vi "Autonomous State Machine.vi"   [LabVIEW 2014]
doc: "This VI is called when autonomous begins, and will automatically be terminated when autonomous ends. You can carry out timed or sensor driven robot movement independently without needing to return to the caller."
uses:
  <vilib>/Rock Robotics/WPI/RobotDrive/WPI_RobotDriveGetSetRefNum.vi
panel:
  # "Be sure to right-click and choose Data Operations>>Make Current Value default if you want to save the array values with the VI"
types:
  T1 = typedef "WPI_MotorControlDeviceRef.ctl" = cluster{"DeviceStatus":errorcluster, "Type":T2, "PWM":cluster{"Controller":T3, "PWM Channel":T4, "DeadBand":T5}, "CAN":cluster{"Device Number":u8, "Control Mode":T6, "Semaphore":T7, "Max Vout":dbl, "TalonSRX Control Mode":T8}, "Invert":bool, "TransformRef":T9, "InvTransformRef":T9}
  T2 = typedef "WPI_MotorControlType.ctl" = enum16{"PWM", "CAN", "CANTalonSRX"}
  T3 = typedef "FPGA_TypedefDigitalModule.ctl" = enum16{"Controller 1"}
  T4 = typedef "FPGA_DIOPWMChannel.ctl" = enum8{"PWM 0", "PWM 1", "PWM 2", "PWM 3", "PWM 4", "PWM 5", "PWM 6", "PWM 7", "PWM 8", "PWM 9", "PWM MXP 0", "PWM MXP 1", "PWM MXP 2", "PWM MXP 3", "PWM MXP 4", "PWM MXP 5", "PWM MXP 6", "PWM MXP 7", "PWM MXP 8", "PWM MXP 9", "Invalid"}
  T5 = typedef "WPI_PWMDeadband.ctl" = cluster{"Name":string, "maxPositivePwm":i32, "minPositivePwm":i32, "centerPwm":i32, "maxNegativePwm":i32, "minNegativePwm":i32, "angularRange":u16}
  T6 = typedef "WPI_CANJaguar_ControlMode.ctl" = enum8{"Percent VBus", "Current", "Speed", "Position", "Voltage"}
  T7 = typedef "Semaphore RefNum" = refnum<k1>
  T8 = typedef "WPI_CANTalonSRX_APIControlMode.ctl" = enum8{"Percent VBus", "Speed", "Position", "Slave", "Unchanged / Invalid"}
  T9 = typedef "WPI_PWMTransform_ConPane.ctl" = refnum<vi>
  T10 = typedef "WPI_DigitalInputDevRef.ctl" = cluster{"DevStatus":errorcluster, "DIO Channel":T11, "Controller":T3}
  T11 = typedef "FPGA_DIOChannel.ctl" = enum8{"DIO 0", "DIO 1", "DIO 2", "DIO 3", "DIO 4", "DIO 5", "DIO 6", "DIO 7", "DIO 8", "DIO 9", "DIO MXP 0", "DIO MXP 1", "DIO MXP 2", "DIO MXP 3", "DIO MXP 4", "DIO MXP 5", "DIO MXP 6", "DIO MXP 7", "DIO MXP 8", "DIO MXP 9", "DIO MXP 10", "DIO MXP 11", "DIO MXP 12", "DIO MXP 13", "DIO MXP 14", "DIO MXP 15", "Invalid"}
  T12 = typedef "WPI_RobotDriveDevRef.ctl" = cluster{"DevStatus":errorcluster, "Motors[]":T1[], "Square Inputs":bool, "Max Output":dbl}
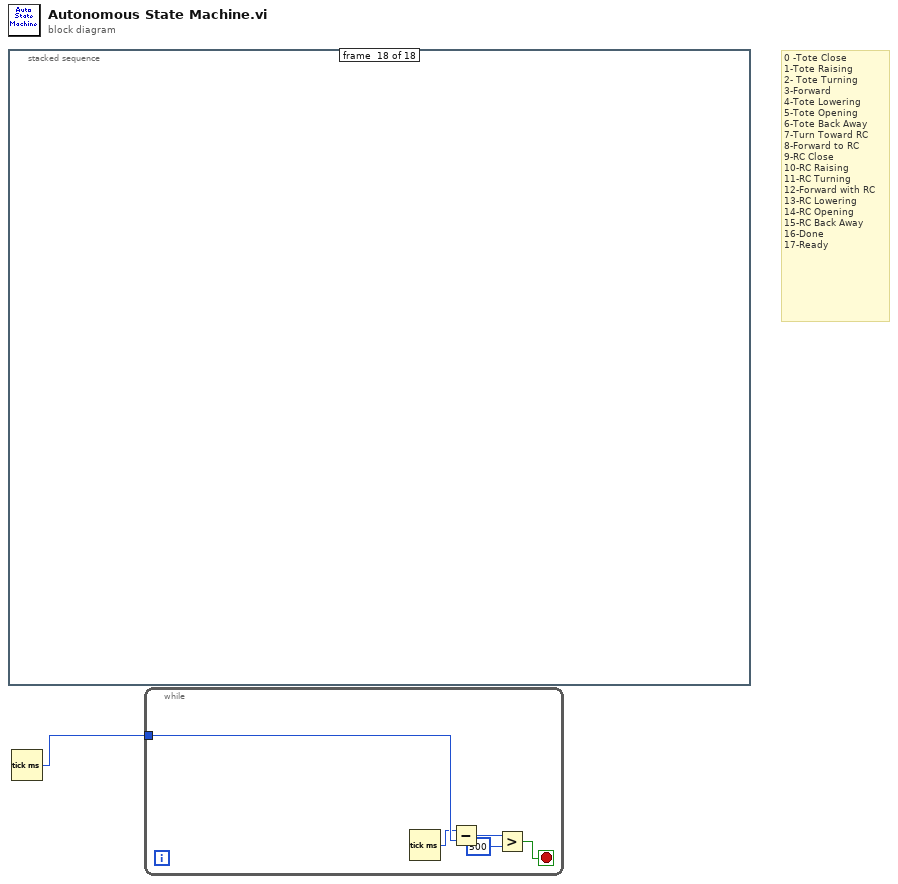
[diagram p0: block diagram]
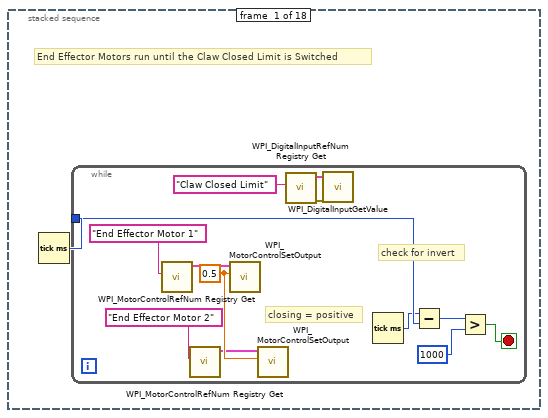
[diagram p2: hidden frame]
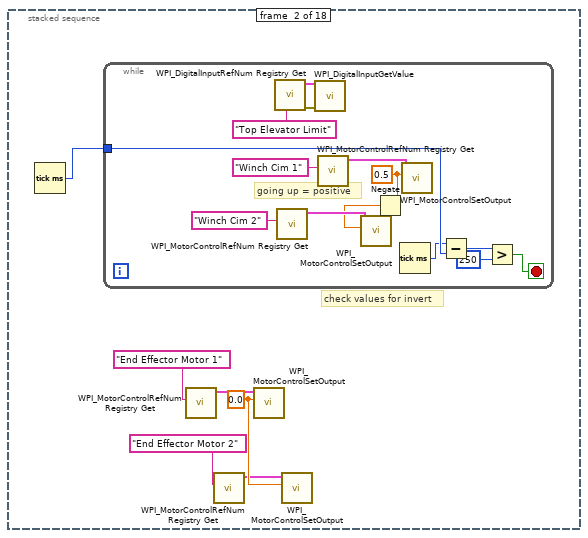
[diagram p3: hidden frame]
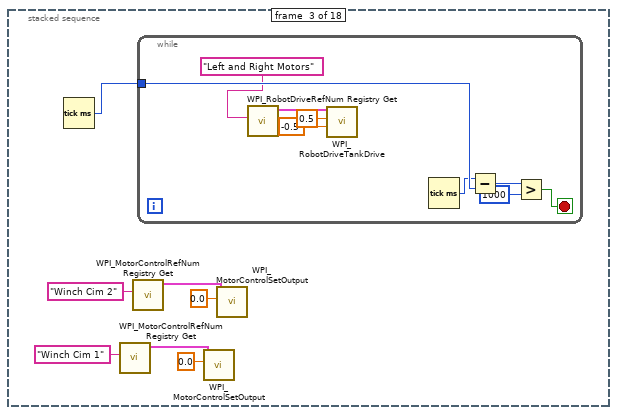
[diagram p4: hidden frame]
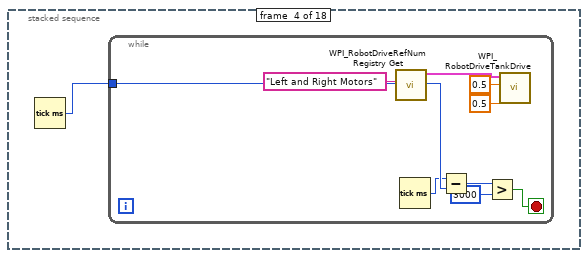
[diagram p5: hidden frame]
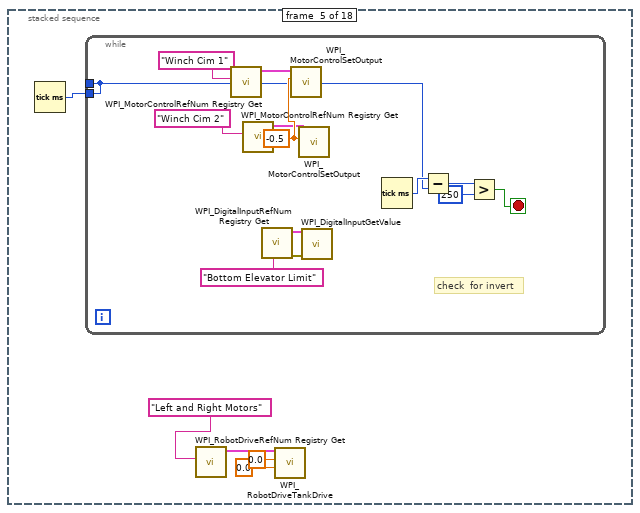
[diagram p6: hidden frame]
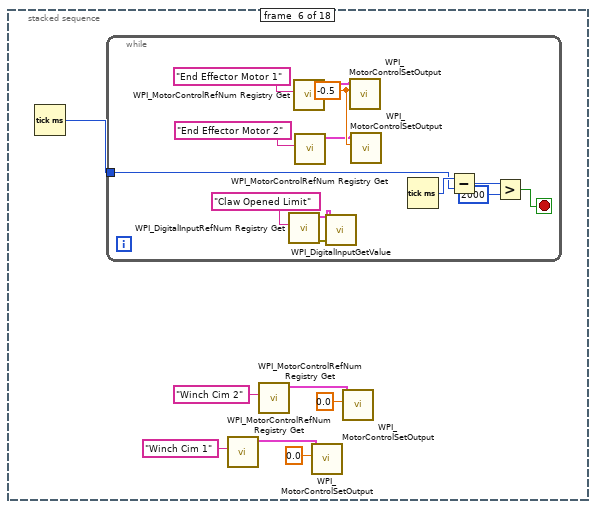
[diagram p7: hidden frame]
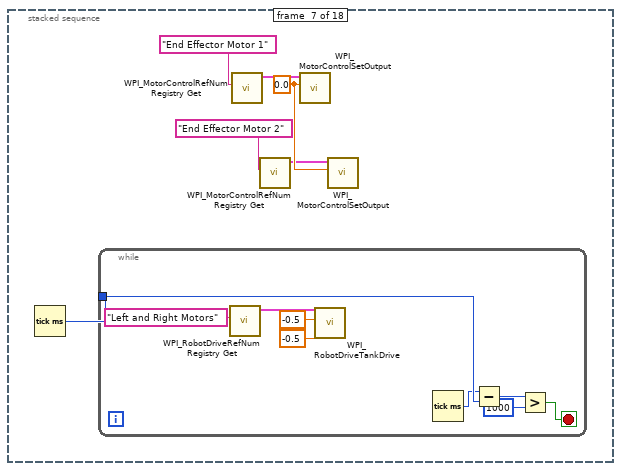
[diagram p8: hidden frame]
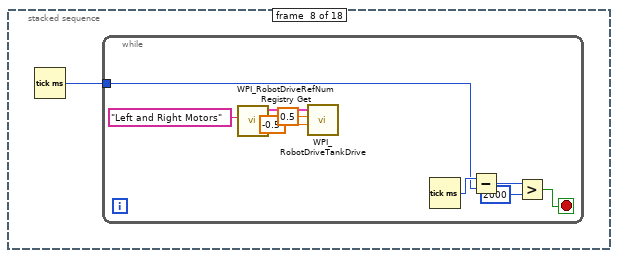
[diagram p9: hidden frame]
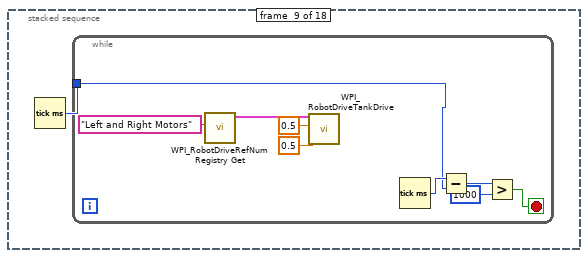
[diagram p10: hidden frame]
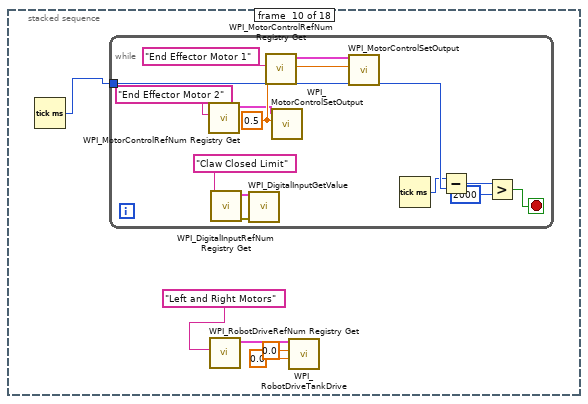
[diagram p11: hidden frame]
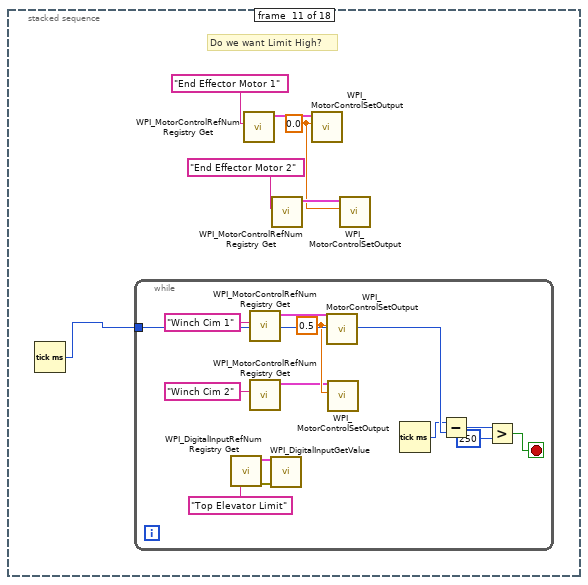
[diagram p12: hidden frame]
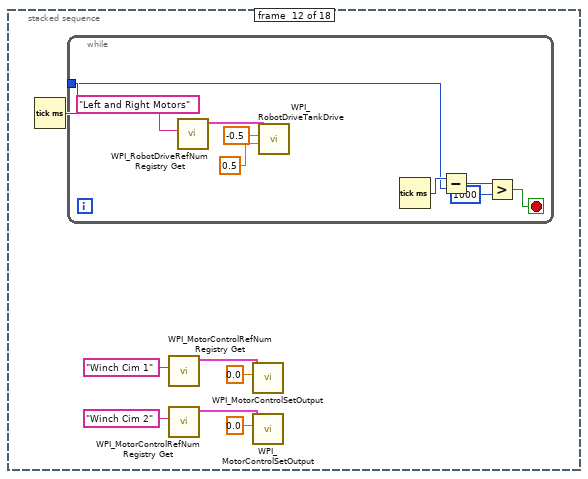
[diagram p13: hidden frame]
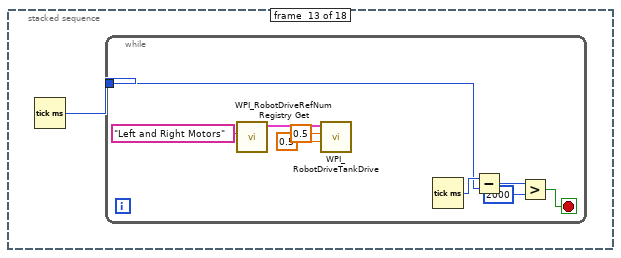
[diagram p14: hidden frame]
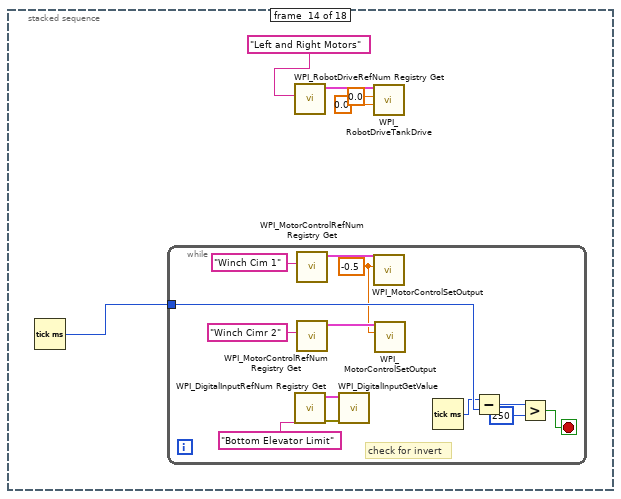
[diagram p15: hidden frame]
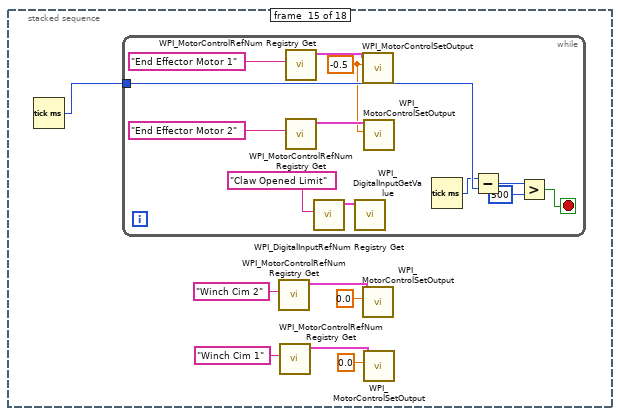
[diagram p16: hidden frame]
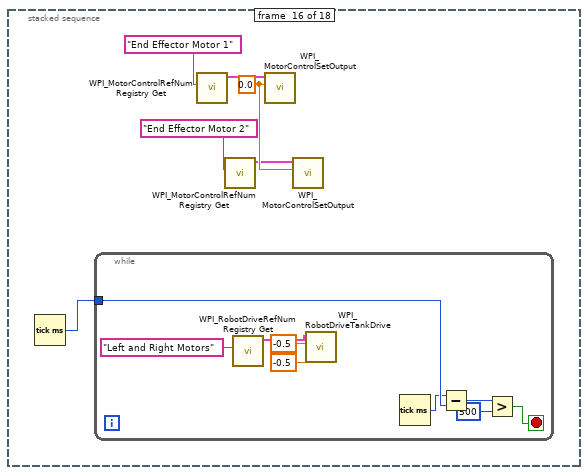
[diagram p17: hidden frame]
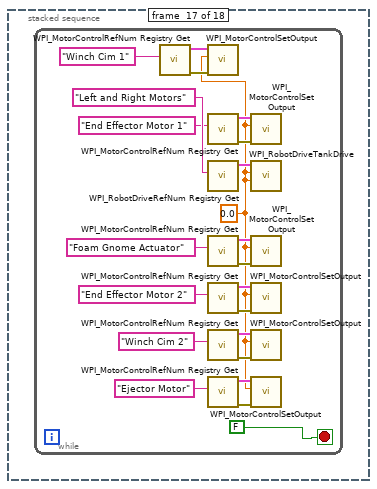
[diagram p18: hidden frame]
diagram:
  # "0 -Tote Close\n1-Tote Raising\n2- Tote Turning\n3-Forward\n4-Tote Lowering\n5-Tote Opening\n6-Tote Back Away\n7-Turn Toward RC\n8-Forward to RC\n9-RC Close\n10-RC Raising\n11-RC Turning\n12-Forward with RC\n13-RC Lowering\n14-RC Opening\n15-RC Back Away\n16-Done\n17-Ready"
  n1 = stacked-sequence {
    frame #0 {
      # "End Effector Motors run until the Claw Closed Limit is Switched"
      n2 = Tick Count (ms)() -> (millisecond timer value=w2:u32)
      n3 = while {
        tunnel: w2 -> [w12]
        stop <- w13 stop-if-true
        w9 = 0.5 ("Output")
        # "closing = positive"
        # "check for invert"
        n4 = call <vilib>:"WPI_MotorControlRefNum Registry Get.vi"("refnum name"="End Effector Motor 1") -> ("MotorControlDevRef"=w6:T1)  [unwired: 9 in, 1 out]
        n5 = call <vilib>:"WPI_MotorControlRefNum Registry Get.vi"("refnum name"="End Effector Motor 2") -> ("MotorControlDevRef"=w8:T1)  [unwired: 9 in, 1 out]
        n6 = call <vilib>:"WPI_MotorControlSetOutput.vi"("Output"=w9, "MotorControlDevRef"=w6) -> ()  [unwired: 7 in, 3 out]
        n7 = call <vilib>:"WPI_MotorControlSetOutput.vi"("Output"=w9, "MotorControlDevRef"=w8) -> ()  [unwired: 7 in, 3 out]
        n8 = call <vilib>:"WPI_DigitalInputRefNum Registry Get.vi"("refnum name"="Claw Closed Limit") -> ("error out"=w4:errorcluster, "DigitalInputDevRef"=w3:T10)  [unwired: 9 in]
        n9 = call <vilib>:"WPI_DigitalInputGetValue.vi"("error in (no error)"=w4, "DigitalInputDevRef"=w3) -> ()  [unwired: 7 in, 3 out]
        n10 = Tick Count (ms)() -> (millisecond timer value=w11:u32)
        n11 = Subtract(x=w11, y=w12) -> (x-y=w15:u32)
        n12 = Greater?(x=w15, y=u32 1000) -> (0:w13:bool)
      }
    }
    frame #1 {
      w19 = 0.0 ("Output")
      # "check values for invert"
      n13 = Tick Count (ms)() -> (millisecond timer value=w21:u32)
      n14 = while {
        tunnel: w21 -> [w26]
        stop <- w27 stop-if-true
        w31 = 0.5 ("Output")
        # "going up = positive"
        n15 = call <vilib>:"WPI_DigitalInputRefNum Registry Get.vi"("refnum name"="Top Elevator Limit") -> ("error out"=w23:errorcluster, "DigitalInputDevRef"=w22:T10)  [unwired: 9 in]
        n16 = call <vilib>:"WPI_MotorControlRefNum Registry Get.vi"("refnum name"="Winch Cim 2") -> ("MotorControlDevRef"=w33:T1)  [unwired: 9 in, 1 out]
        n17 = call <vilib>:"WPI_DigitalInputGetValue.vi"("error in (no error)"=w23, "DigitalInputDevRef"=w22) -> ()  [unwired: 7 in, 3 out]
        n18 = call <vilib>:"WPI_MotorControlRefNum Registry Get.vi"("refnum name"="Winch Cim 1") -> ("MotorControlDevRef"=w35:T1)  [unwired: 9 in, 1 out]
        n19 = Negate(x=w31) -> (-x=w30:dbl)
        n20 = call <vilib>:"WPI_MotorControlSetOutput.vi"("Output"=w30, "MotorControlDevRef"=w33) -> ()  [unwired: 7 in, 3 out]
        n21 = Tick Count (ms)() -> (millisecond timer value=w25:u32)
        n22 = call <vilib>:"WPI_MotorControlSetOutput.vi"("Output"=w31, "MotorControlDevRef"=w35) -> ()  [unwired: 7 in, 3 out]
        n23 = Subtract(x=w25, y=w26) -> (x-y=w29:u32)
        n24 = Greater?(x=w29, y=u32 250) -> (0:w27:bool)
      }
      n25 = call <vilib>:"WPI_MotorControlRefNum Registry Get.vi"("refnum name"="End Effector Motor 1") -> ("MotorControlDevRef"=w16:T1)  [unwired: 9 in, 1 out]
      n26 = call <vilib>:"WPI_MotorControlRefNum Registry Get.vi"("refnum name"="End Effector Motor 2") -> ("MotorControlDevRef"=w18:T1)  [unwired: 9 in, 1 out]
      n27 = call <vilib>:"WPI_MotorControlSetOutput.vi"("Output"=w19, "MotorControlDevRef"=w16) -> ()  [unwired: 7 in, 3 out]
      n28 = call <vilib>:"WPI_MotorControlSetOutput.vi"("Output"=w19, "MotorControlDevRef"=w18) -> ()  [unwired: 7 in, 3 out]
    }
    frame #2 {
      n29 = Tick Count (ms)() -> (millisecond timer value=w42:u32)
      n30 = call <vilib>:"WPI_MotorControlRefNum Registry Get.vi"("refnum name"="Winch Cim 1") -> ("MotorControlDevRef"=w37:T1)  [unwired: 9 in, 1 out]
      n31 = call <vilib>:"WPI_MotorControlRefNum Registry Get.vi"("refnum name"="Winch Cim 2") -> ("MotorControlDevRef"=w40:T1)  [unwired: 9 in, 1 out]
      n32 = while {
        tunnel: w42 -> [w48]
        stop <- w49 stop-if-true
        n33 = call <vilib>:"WPI_RobotDriveRefNum Registry Get.vi"("refnum name"="Left and Right Motors") -> ("RobotDriveDevRef"=w46:T12)  [unwired: 9 in, 1 out]
        n34 = call <vilib>:"WPI_RobotDriveTankDrive.vi"("Right axis value"=-0.5, "Left axis value"=0.5, "RobotDriveDevRef"=w46) -> ()  [unwired: 6 in, 3 out]
        n35 = Tick Count (ms)() -> (millisecond timer value=w47:u32)
        n36 = Subtract(x=w47, y=w48) -> (x-y=w51:u32)
        n37 = Greater?(x=w51, y=u32 1000) -> (0:w49:bool)
      }
      n38 = call <vilib>:"WPI_MotorControlSetOutput.vi"("Output"=0.0, "MotorControlDevRef"=w37) -> ()  [unwired: 7 in, 3 out]
      n39 = call <vilib>:"WPI_MotorControlSetOutput.vi"("Output"=0.0, "MotorControlDevRef"=w40) -> ()  [unwired: 7 in, 3 out]
    }
    frame #3 {
      n40 = Tick Count (ms)() -> (millisecond timer value=w52:u32)
      n41 = while {
        tunnel: w52 -> [w58]
        stop <- w59 stop-if-true
        n42 = call <vilib>:"WPI_RobotDriveRefNum Registry Get.vi"("refnum name"="Left and Right Motors") -> ("RobotDriveDevRef"=w56:T12)  [unwired: 9 in, 1 out]
        n43 = Tick Count (ms)() -> (millisecond timer value=w57:u32)
        n44 = Subtract(x=w57, y=w58) -> (x-y=w61:u32)
        n45 = Greater?(x=w61, y=u32 3000) -> (0:w59:bool)
        n46 = call <vilib>:"WPI_RobotDriveTankDrive.vi"("Right axis value"=0.5, "Left axis value"=0.5, "RobotDriveDevRef"=w56) -> ()  [unwired: 6 in, 3 out]
      }
    }
    frame #4 {
      n47 = Tick Count (ms)() -> (millisecond timer value=w66:u32)
      n48 = while {
        tunnel: [w70] -> _
        tunnel: w66 -> [w70]
        stop <- w77 stop-if-true
        w75 = -0.5 ("Output")
        # "check  for invert"
        n49 = call <vilib>:"WPI_MotorControlRefNum Registry Get.vi"("refnum name"="Winch Cim 1") -> ("MotorControlDevRef"=w73:T1)  [unwired: 9 in, 1 out]
        n50 = call <vilib>:"WPI_MotorControlRefNum Registry Get.vi"("refnum name"="Winch Cim 2") -> ("MotorControlDevRef"=w74:T1)  [unwired: 9 in, 1 out]
        n51 = call <vilib>:"WPI_DigitalInputRefNum Registry Get.vi"("refnum name"="Bottom Elevator Limit") -> ("error out"=w68:errorcluster, "DigitalInputDevRef"=w67:T10)  [unwired: 9 in]
        n52 = call <vilib>:"WPI_MotorControlSetOutput.vi"("Output"=w75, "MotorControlDevRef"=w73) -> ()  [unwired: 7 in, 3 out]
        n53 = call <vilib>:"WPI_MotorControlSetOutput.vi"("Output"=w75, "MotorControlDevRef"=w74) -> ()  [unwired: 7 in, 3 out]
        n54 = call <vilib>:"WPI_DigitalInputGetValue.vi"("error in (no error)"=w68, "DigitalInputDevRef"=w67) -> ()  [unwired: 7 in, 3 out]
        n55 = Tick Count (ms)() -> (millisecond timer value=w76:u32)
        n56 = Subtract(x=w76, y=w70) -> (x-y=w79:u32)
        n57 = Greater?(x=w79, y=u32 250) -> (0:w77:bool)
      }
      n58 = call <vilib>:"WPI_RobotDriveRefNum Registry Get.vi"("refnum name"="Left and Right Motors") -> ("RobotDriveDevRef"=w65:T12)  [unwired: 9 in, 1 out]
      n59 = call <vilib>:"WPI_RobotDriveTankDrive.vi"("Right axis value"=0.0, "Left axis value"=0.0, "RobotDriveDevRef"=w65) -> ()  [unwired: 6 in, 3 out]
    }
    frame #5 {
      n60 = Tick Count (ms)() -> (millisecond timer value=w86:u32)
      n61 = while {
        tunnel: w86 -> [w90]
        stop <- w97 stop-if-true
        w95 = -0.5 ("Output")
        n62 = call <vilib>:"WPI_DigitalInputRefNum Registry Get.vi"("refnum name"="Claw Opened Limit") -> ("error out"=w88:errorcluster, "DigitalInputDevRef"=w89:T10)  [unwired: 9 in]
        n63 = call <vilib>:"WPI_MotorControlRefNum Registry Get.vi"("refnum name"="End Effector Motor 1") -> ("MotorControlDevRef"=w92:T1)  [unwired: 9 in, 1 out]
        n64 = call <vilib>:"WPI_MotorControlRefNum Registry Get.vi"("refnum name"="End Effector Motor 2") -> ("MotorControlDevRef"=w94:T1)  [unwired: 9 in, 1 out]
        n65 = call <vilib>:"WPI_DigitalInputGetValue.vi"("error in (no error)"=w88, "DigitalInputDevRef"=w89) -> ()  [unwired: 7 in, 3 out]
        n66 = call <vilib>:"WPI_MotorControlSetOutput.vi"("Output"=w95, "MotorControlDevRef"=w92) -> ()  [unwired: 7 in, 3 out]
        n67 = call <vilib>:"WPI_MotorControlSetOutput.vi"("Output"=w95, "MotorControlDevRef"=w94) -> ()  [unwired: 7 in, 3 out]
        n68 = Tick Count (ms)() -> (millisecond timer value=w96:u32)
        n69 = Subtract(x=w96, y=w90) -> (x-y=w99:u32)
        n70 = Greater?(x=w99, y=u32 2000) -> (0:w97:bool)
      }
      n71 = call <vilib>:"WPI_MotorControlRefNum Registry Get.vi"("refnum name"="Winch Cim 1") -> ("MotorControlDevRef"=w81:T1)  [unwired: 9 in, 1 out]
      n72 = call <vilib>:"WPI_MotorControlRefNum Registry Get.vi"("refnum name"="Winch Cim 2") -> ("MotorControlDevRef"=w84:T1)  [unwired: 9 in, 1 out]
      n73 = call <vilib>:"WPI_MotorControlSetOutput.vi"("Output"=0.0, "MotorControlDevRef"=w81) -> ()  [unwired: 7 in, 3 out]
      n74 = call <vilib>:"WPI_MotorControlSetOutput.vi"("Output"=0.0, "MotorControlDevRef"=w84) -> ()  [unwired: 7 in, 3 out]
    }
    frame #6 {
      w103 = 0.0 ("Output")
      n75 = Tick Count (ms)() -> (millisecond timer value=w105:u32)
      n76 = while {
        tunnel: w105 -> [w111]
        stop <- w112 stop-if-true
        n77 = call <vilib>:"WPI_RobotDriveRefNum Registry Get.vi"("refnum name"="Left and Right Motors") -> ("RobotDriveDevRef"=w109:T12)  [unwired: 9 in, 1 out]
        n78 = call <vilib>:"WPI_RobotDriveTankDrive.vi"("Right axis value"=-0.5, "Left axis value"=-0.5, "RobotDriveDevRef"=w109) -> ()  [unwired: 6 in, 3 out]
        n79 = Tick Count (ms)() -> (millisecond timer value=w110:u32)
        n80 = Subtract(x=w110, y=w111) -> (x-y=w114:u32)
        n81 = Greater?(x=w114, y=u32 1000) -> (0:w112:bool)
      }
      n82 = call <vilib>:"WPI_MotorControlRefNum Registry Get.vi"("refnum name"="End Effector Motor 1") -> ("MotorControlDevRef"=w100:T1)  [unwired: 9 in, 1 out]
      n83 = call <vilib>:"WPI_MotorControlRefNum Registry Get.vi"("refnum name"="End Effector Motor 2") -> ("MotorControlDevRef"=w102:T1)  [unwired: 9 in, 1 out]
      n84 = call <vilib>:"WPI_MotorControlSetOutput.vi"("Output"=w103, "MotorControlDevRef"=w100) -> ()  [unwired: 7 in, 3 out]
      n85 = call <vilib>:"WPI_MotorControlSetOutput.vi"("Output"=w103, "MotorControlDevRef"=w102) -> ()  [unwired: 7 in, 3 out]
    }
    frame #7 {
      n86 = Tick Count (ms)() -> (millisecond timer value=w115:u32)
      n87 = while {
        tunnel: w115 -> [w120]
        stop <- w122 stop-if-true
        n88 = call <vilib>:"WPI_RobotDriveRefNum Registry Get.vi"("refnum name"="Left and Right Motors") -> ("RobotDriveDevRef"=w119:T12)  [unwired: 9 in, 1 out]
        n89 = call <vilib>:"WPI_RobotDriveTankDrive.vi"("Right axis value"=-0.5, "Left axis value"=0.5, "RobotDriveDevRef"=w119) -> ()  [unwired: 6 in, 3 out]
        n90 = Tick Count (ms)() -> (millisecond timer value=w121:u32)
        n91 = Subtract(x=w121, y=w120) -> (x-y=w124:u32)
        n92 = Greater?(x=w124, y=u32 2000) -> (0:w122:bool)
      }
    }
    frame #8 {
      n93 = Tick Count (ms)() -> (millisecond timer value=w125:u32)
      n94 = while {
        tunnel: w125 -> [w130]
        stop <- w132 stop-if-true
        n95 = call <vilib>:"WPI_RobotDriveRefNum Registry Get.vi"("refnum name"="Left and Right Motors") -> ("RobotDriveDevRef"=w129:T12)  [unwired: 9 in, 1 out]
        n96 = call <vilib>:"WPI_RobotDriveTankDrive.vi"("Right axis value"=0.5, "Left axis value"=0.5, "RobotDriveDevRef"=w129) -> ()  [unwired: 6 in, 3 out]
        n97 = Tick Count (ms)() -> (millisecond timer value=w131:u32)
        n98 = Subtract(x=w131, y=w130) -> (x-y=w134:u32)
        n99 = Greater?(x=w134, y=u32 1000) -> (0:w132:bool)
      }
    }
    frame #9 {
      n100 = Tick Count (ms)() -> (millisecond timer value=w139:u32)
      n101 = while {
        tunnel: w139 -> [w149]
        stop <- w150 stop-if-true
        w147 = 0.5 ("Output")
        n102 = call <vilib>:"WPI_MotorControlRefNum Registry Get.vi"("refnum name"="End Effector Motor 2") -> ("MotorControlDevRef"=w144:T1)  [unwired: 9 in, 1 out]
        n103 = call <vilib>:"WPI_DigitalInputRefNum Registry Get.vi"("refnum name"="Claw Closed Limit") -> ("error out"=w141:errorcluster, "DigitalInputDevRef"=w142:T10)  [unwired: 9 in]
        n104 = call <vilib>:"WPI_DigitalInputGetValue.vi"("error in (no error)"=w141, "DigitalInputDevRef"=w142) -> ()  [unwired: 7 in, 3 out]
        n105 = call <vilib>:"WPI_MotorControlRefNum Registry Get.vi"("refnum name"="End Effector Motor 1") -> ("MotorControlDevRef"=w143:T1)  [unwired: 9 in, 1 out]
        n106 = call <vilib>:"WPI_MotorControlSetOutput.vi"("Output"=w147, "MotorControlDevRef"=w144) -> ()  [unwired: 7 in, 3 out]
        n107 = call <vilib>:"WPI_MotorControlSetOutput.vi"("Output"=w147, "MotorControlDevRef"=w143) -> ()  [unwired: 7 in, 3 out]
        n108 = Tick Count (ms)() -> (millisecond timer value=w148:u32)
        n109 = Subtract(x=w148, y=w149) -> (x-y=w152:u32)
        n110 = Greater?(x=w152, y=u32 2000) -> (0:w150:bool)
      }
      n111 = call <vilib>:"WPI_RobotDriveRefNum Registry Get.vi"("refnum name"="Left and Right Motors") -> ("RobotDriveDevRef"=w138:T12)  [unwired: 9 in, 1 out]
      n112 = call <vilib>:"WPI_RobotDriveTankDrive.vi"("Right axis value"=0.0, "Left axis value"=0.0, "RobotDriveDevRef"=w138) -> ()  [unwired: 6 in, 3 out]
    }
    frame #10 {
      w154 = 0.0 ("Output")
      # "Do we want Limit High?"
      n113 = Tick Count (ms)() -> (millisecond timer value=w158:u32)
      n114 = while {
        tunnel: w158 -> [w168]
        stop <- w169 stop-if-true
        w166 = 0.5 ("Output")
        n115 = call <vilib>:"WPI_DigitalInputRefNum Registry Get.vi"("refnum name"="Top Elevator Limit") -> ("error out"=w160:errorcluster, "DigitalInputDevRef"=w159:T10)  [unwired: 9 in]
        n116 = call <vilib>:"WPI_MotorControlRefNum Registry Get.vi"("refnum name"="Winch Cim 1") -> ("MotorControlDevRef"=w162:T1)  [unwired: 9 in, 1 out]
        n117 = call <vilib>:"WPI_MotorControlRefNum Registry Get.vi"("refnum name"="Winch Cim 2") -> ("MotorControlDevRef"=w163:T1)  [unwired: 9 in, 1 out]
        n118 = call <vilib>:"WPI_DigitalInputGetValue.vi"("error in (no error)"=w160, "DigitalInputDevRef"=w159) -> ()  [unwired: 7 in, 3 out]
        n119 = call <vilib>:"WPI_MotorControlSetOutput.vi"("Output"=w166, "MotorControlDevRef"=w162) -> ()  [unwired: 7 in, 3 out]
        n120 = call <vilib>:"WPI_MotorControlSetOutput.vi"("Output"=w166, "MotorControlDevRef"=w163) -> ()  [unwired: 7 in, 3 out]
        n121 = Tick Count (ms)() -> (millisecond timer value=w167:u32)
        n122 = Subtract(x=w167, y=w168) -> (x-y=w171:u32)
        n123 = Greater?(x=w171, y=u32 250) -> (0:w169:bool)
      }
      n124 = call <vilib>:"WPI_MotorControlRefNum Registry Get.vi"("refnum name"="End Effector Motor 1") -> ("MotorControlDevRef"=w157:T1)  [unwired: 9 in, 1 out]
      n125 = call <vilib>:"WPI_MotorControlRefNum Registry Get.vi"("refnum name"="End Effector Motor 2") -> ("MotorControlDevRef"=w155:T1)  [unwired: 9 in, 1 out]
      n126 = call <vilib>:"WPI_MotorControlSetOutput.vi"("Output"=w154, "MotorControlDevRef"=w157) -> ()  [unwired: 7 in, 3 out]
      n127 = call <vilib>:"WPI_MotorControlSetOutput.vi"("Output"=w154, "MotorControlDevRef"=w155) -> ()  [unwired: 7 in, 3 out]
    }
    frame #11 {
      n128 = Tick Count (ms)() -> (millisecond timer value=w178:u32)
      n129 = while {
        tunnel: w178 -> [w183]
        stop <- w185 stop-if-true
        n130 = call <vilib>:"WPI_RobotDriveRefNum Registry Get.vi"("refnum name"="Left and Right Motors") -> ("RobotDriveDevRef"=w182:T12)  [unwired: 9 in, 1 out]
        n131 = call <vilib>:"WPI_RobotDriveTankDrive.vi"("Right axis value"=0.5, "Left axis value"=-0.5, "RobotDriveDevRef"=w182) -> ()  [unwired: 6 in, 3 out]
        n132 = Tick Count (ms)() -> (millisecond timer value=w184:u32)
        n133 = Subtract(x=w184, y=w183) -> (x-y=w187:u32)
        n134 = Greater?(x=w187, y=u32 1000) -> (0:w185:bool)
      }
      n135 = call <vilib>:"WPI_MotorControlRefNum Registry Get.vi"("refnum name"="Winch Cim 1") -> ("MotorControlDevRef"=w176:T1)  [unwired: 9 in, 1 out]
      n136 = call <vilib>:"WPI_MotorControlRefNum Registry Get.vi"("refnum name"="Winch Cim 2") -> ("MotorControlDevRef"=w173:T1)  [unwired: 9 in, 1 out]
      n137 = call <vilib>:"WPI_MotorControlSetOutput.vi"("Output"=0.0, "MotorControlDevRef"=w176) -> ()  [unwired: 7 in, 3 out]
      n138 = call <vilib>:"WPI_MotorControlSetOutput.vi"("Output"=0.0, "MotorControlDevRef"=w173) -> ()  [unwired: 7 in, 3 out]
    }
    frame #12 {
      n139 = Tick Count (ms)() -> (millisecond timer value=w188:u32)
      n140 = while {
        tunnel: w188 -> [w193]
        stop <- w195 stop-if-true
        n141 = call <vilib>:"WPI_RobotDriveRefNum Registry Get.vi"("refnum name"="Left and Right Motors") -> ("RobotDriveDevRef"=w192:T12)  [unwired: 9 in, 1 out]
        n142 = call <vilib>:"WPI_RobotDriveTankDrive.vi"("Right axis value"=0.5, "Left axis value"=0.5, "RobotDriveDevRef"=w192) -> ()  [unwired: 6 in, 3 out]
        n143 = Tick Count (ms)() -> (millisecond timer value=w194:u32)
        n144 = Subtract(x=w194, y=w193) -> (x-y=w197:u32)
        n145 = Greater?(x=w197, y=u32 2000) -> (0:w195:bool)
      }
    }
    frame #13 {
      n146 = Tick Count (ms)() -> (millisecond timer value=w202:u32)
      n147 = while {
        tunnel: w202 -> [w212]
        stop <- w213 stop-if-true
        w203 = -0.5 ("Output")
        # "check for invert"
        n148 = call <vilib>:"WPI_DigitalInputRefNum Registry Get.vi"("refnum name"="Bottom Elevator Limit") -> ("error out"=w209:errorcluster, "DigitalInputDevRef"=w208:T10)  [unwired: 9 in]
        n149 = call <vilib>:"WPI_MotorControlRefNum Registry Get.vi"("refnum name"="Winch Cim 1") -> ("MotorControlDevRef"=w207:T1)  [unwired: 9 in, 1 out]
        n150 = call <vilib>:"WPI_MotorControlRefNum Registry Get.vi"("refnum name"="Winch Cimr 2") -> ("MotorControlDevRef"=w206:T1)  [unwired: 9 in, 1 out]
        n151 = call <vilib>:"WPI_DigitalInputGetValue.vi"("error in (no error)"=w209, "DigitalInputDevRef"=w208) -> ()  [unwired: 7 in, 3 out]
        n152 = call <vilib>:"WPI_MotorControlSetOutput.vi"("Output"=w203, "MotorControlDevRef"=w207) -> ()  [unwired: 7 in, 3 out]
        n153 = call <vilib>:"WPI_MotorControlSetOutput.vi"("Output"=w203, "MotorControlDevRef"=w206) -> ()  [unwired: 7 in, 3 out]
        n154 = Tick Count (ms)() -> (millisecond timer value=w211:u32)
        n155 = Subtract(x=w211, y=w212) -> (x-y=w215:u32)
        n156 = Greater?(x=w215, y=u32 250) -> (0:w213:bool)
      }
      n157 = call <vilib>:"WPI_RobotDriveRefNum Registry Get.vi"("refnum name"="Left and Right Motors") -> ("RobotDriveDevRef"=w201:T12)  [unwired: 9 in, 1 out]
      n158 = call <vilib>:"WPI_RobotDriveTankDrive.vi"("Right axis value"=0.0, "Left axis value"=0.0, "RobotDriveDevRef"=w201) -> ()  [unwired: 6 in, 3 out]
    }
    frame #14 {
      n159 = Tick Count (ms)() -> (millisecond timer value=w222:u32)
      n160 = while {
        tunnel: w222 -> [w231]
        stop <- w232 stop-if-true
        w224 = -0.5 ("Output")
        n161 = call <vilib>:"WPI_MotorControlRefNum Registry Get.vi"("refnum name"="End Effector Motor 1") -> ("MotorControlDevRef"=w223:T1)  [unwired: 9 in, 1 out]
        n162 = call <vilib>:"WPI_MotorControlRefNum Registry Get.vi"("refnum name"="End Effector Motor 2") -> ("MotorControlDevRef"=w227:T1)  [unwired: 9 in, 1 out]
        n163 = call <vilib>:"WPI_DigitalInputRefNum Registry Get.vi"("refnum name"="Claw Opened Limit") -> ("DigitalInputDevRef"=w228:T10)  [unwired: 9 in, 1 out]
        n164 = call <vilib>:"WPI_DigitalInputGetValue.vi"("DigitalInputDevRef"=w228) -> ()  [unwired: 8 in, 3 out]
        n165 = call <vilib>:"WPI_MotorControlSetOutput.vi"("Output"=w224, "MotorControlDevRef"=w223) -> ()  [unwired: 7 in, 3 out]
        n166 = call <vilib>:"WPI_MotorControlSetOutput.vi"("Output"=w224, "MotorControlDevRef"=w227) -> ()  [unwired: 7 in, 3 out]
        n167 = Tick Count (ms)() -> (millisecond timer value=w230:u32)
        n168 = Subtract(x=w230, y=w231) -> (x-y=w234:u32)
        n169 = Greater?(x=w234, y=u32 500) -> (0:w232:bool)
      }
      n170 = call <vilib>:"WPI_MotorControlRefNum Registry Get.vi"("refnum name"="Winch Cim 2") -> ("MotorControlDevRef"=w220:T1)  [unwired: 9 in, 1 out]
      n171 = call <vilib>:"WPI_MotorControlRefNum Registry Get.vi"("refnum name"="Winch Cim 1") -> ("MotorControlDevRef"=w217:T1)  [unwired: 9 in, 1 out]
      n172 = call <vilib>:"WPI_MotorControlSetOutput.vi"("Output"=0.0, "MotorControlDevRef"=w220) -> ()  [unwired: 7 in, 3 out]
      n173 = call <vilib>:"WPI_MotorControlSetOutput.vi"("Output"=0.0, "MotorControlDevRef"=w217) -> ()  [unwired: 7 in, 3 out]
    }
    frame #15 {
      w238 = 0.0 ("Output")
      n174 = Tick Count (ms)() -> (millisecond timer value=w240:u32)
      n175 = while {
        tunnel: w240 -> [w246]
        stop <- w247 stop-if-true
        n176 = call <vilib>:"WPI_RobotDriveRefNum Registry Get.vi"("refnum name"="Left and Right Motors") -> ("RobotDriveDevRef"=w244:T12)  [unwired: 9 in, 1 out]
        n177 = call <vilib>:"WPI_RobotDriveTankDrive.vi"("Right axis value"=-0.5, "Left axis value"=-0.5, "RobotDriveDevRef"=w244) -> ()  [unwired: 6 in, 3 out]
        n178 = Tick Count (ms)() -> (millisecond timer value=w245:u32)
        n179 = Subtract(x=w245, y=w246) -> (x-y=w249:u32)
        n180 = Greater?(x=w249, y=u32 500) -> (0:w247:bool)
      }
      n181 = call <vilib>:"WPI_MotorControlRefNum Registry Get.vi"("refnum name"="End Effector Motor 1") -> ("MotorControlDevRef"=w235:T1)  [unwired: 9 in, 1 out]
      n182 = call <vilib>:"WPI_MotorControlRefNum Registry Get.vi"("refnum name"="End Effector Motor 2") -> ("MotorControlDevRef"=w237:T1)  [unwired: 9 in, 1 out]
      n183 = call <vilib>:"WPI_MotorControlSetOutput.vi"("Output"=w238, "MotorControlDevRef"=w235) -> ()  [unwired: 7 in, 3 out]
      n184 = call <vilib>:"WPI_MotorControlSetOutput.vi"("Output"=w238, "MotorControlDevRef"=w237) -> ()  [unwired: 7 in, 3 out]
    }
    frame #16 {
      n185 = while {
        stop <- FALSE stop-if-true
        w251 = 0.0
        n186 = call <vilib>:"WPI_MotorControlRefNum Registry Get.vi"("refnum name"="Winch Cim 1") -> ("error out"=w260:errorcluster, "MotorControlDevRef"=w259:T1)  [unwired: 9 in]
        n187 = call <vilib>:"WPI_MotorControlSetOutput.vi"("error in (no error)"=w260, "Output"=w251, "MotorControlDevRef"=w259) -> ()  [unwired: 6 in, 3 out]
        n188 = call <vilib>:"WPI_MotorControlRefNum Registry Get.vi"("refnum name"="End Effector Motor 1") -> ("error out"=w268:errorcluster, "MotorControlDevRef"=w267:T1)  [unwired: 9 in]
        n189 = call <vilib>:"WPI_RobotDriveRefNum Registry Get.vi"("refnum name"="Left and Right Motors") -> ("RobotDriveDevRef"=w270:T12)  [unwired: 9 in, 1 out]
        n190 = call <vilib>:"WPI_MotorControlRefNum Registry Get.vi"("refnum name"="Foam Gnome Actuator") -> ("error out"=w264:errorcluster, "MotorControlDevRef"=w263:T1)  [unwired: 9 in]
        n191 = call <vilib>:"WPI_MotorControlRefNum Registry Get.vi"("refnum name"="End Effector Motor 2") -> ("error out"=w266:errorcluster, "MotorControlDevRef"=w265:T1)  [unwired: 9 in]
        n192 = call <vilib>:"WPI_MotorControlRefNum Registry Get.vi"("refnum name"="Winch Cim 2") -> ("error out"=w262:errorcluster, "MotorControlDevRef"=w261:T1)  [unwired: 9 in]
        n193 = call <vilib>:"WPI_MotorControlRefNum Registry Get.vi"("refnum name"="Ejector Motor") -> ("error out"=w255:errorcluster, "MotorControlDevRef"=w254:T1)  [unwired: 9 in]
        n194 = call <vilib>:"WPI_MotorControlSetOutput.vi"("error in (no error)"=w268, "Output"=w251, "MotorControlDevRef"=w267) -> ()  [unwired: 6 in, 3 out]
        n195 = call <vilib>:"WPI_RobotDriveTankDrive.vi"("Right axis value"=w251, "Left axis value"=w251, "RobotDriveDevRef"=w270) -> ()  [unwired: 6 in, 3 out]
        n196 = call <vilib>:"WPI_MotorControlSetOutput.vi"("error in (no error)"=w264, "Output"=w251, "MotorControlDevRef"=w263) -> ()  [unwired: 6 in, 3 out]
        n197 = call <vilib>:"WPI_MotorControlSetOutput.vi"("error in (no error)"=w266, "Output"=w251, "MotorControlDevRef"=w265) -> ()  [unwired: 6 in, 3 out]
        n198 = call <vilib>:"WPI_MotorControlSetOutput.vi"("error in (no error)"=w262, "Output"=w251, "MotorControlDevRef"=w261) -> ()  [unwired: 6 in, 3 out]
        n199 = call <vilib>:"WPI_MotorControlSetOutput.vi"("error in (no error)"=w255, "Output"=w251, "MotorControlDevRef"=w254) -> ()  [unwired: 6 in, 3 out]
      }
    }
    frame #17 {
    }
  }
  n200 = Tick Count (ms)() -> (millisecond timer value=w1:u32)
  n201 = while {
    tunnel: w1 -> [w273]
    stop <- w274 stop-if-true
    n202 = Tick Count (ms)() -> (millisecond timer value=w272:u32)
    n203 = Subtract(x=w272, y=w273) -> (x-y=w276:u32)
    n204 = Greater?(x=w276, y=u32 500) -> (0:w274:bool)
  }
